vi "list_documents.vi"(0 "Device In":T1, 5 "error in":errorcluster) -> (14 "Device Out":T1, 15 "Comm":T2, 18 "Document list":string[][](array[string]), 19 "error out":errorcluster)   [LabVIEW 2019]
uses:
  <userlib>/IoT Devices/_subVIs/HTTPComm.ctl
  _SubVI/Cluster.ctl
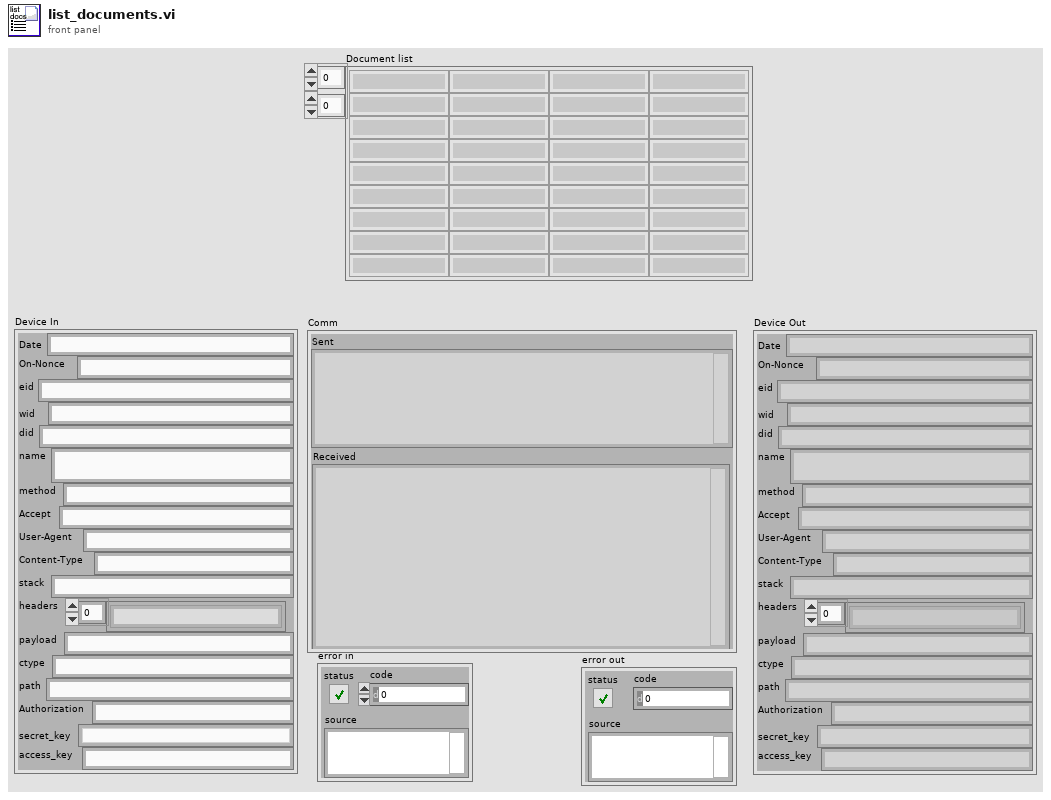
[diagram p1: front panel]
types:
  T1 = typedef "Cluster.ctl" = cluster{"Date":string, "On-Nonce":string, "eid":string, "wid":string, "did":string, "name":string, "method":string, "Accept":string, "User-Agent":string, "Content-Type":string, "stack":string, "headers":string[], "payload":string, "ctype":string, "path":string, "Authorization":string, "secret_key":string, "access_key":string}
  T2 = typedef "HTTPComm.ctl" = cluster{"url":string, "sent headers":string, "sent body":string, "headers":string, "body":string, "Sent":string, "Received":string}
  T3 = cluster{"items":cluster{"resourceType":string, "id":string, "name":string, "defaultWorkspace":cluster{"id":string}}[]}
  T4 = cluster{"resourceType":string, "id":string, "name":string, "defaultWorkspace":cluster{"id":string}}[]
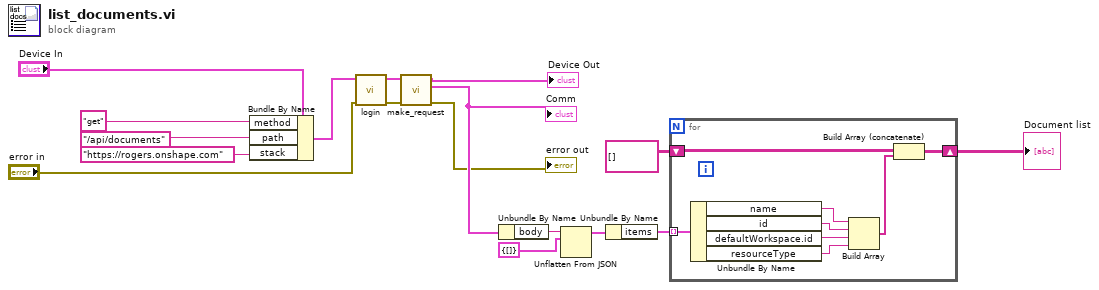
[diagram p0: block diagram]
diagram:
  n1 = Bundle By Name(cluster="Device In", "method"="get" ("Method"), "path"="/api/documents" ("payload"), "stack"="https://rogers.onshape.com" ("stacks")) -> (w5:T1)
  n2 = call "login.vi"("error in"="error in", "Device In"=w5) -> ("error out"=w6:errorcluster, "Device Out"=w4:T1)  [unwired: 8 in]
  n3 = call "make_request.vi"("Error in"=w6, "Device In"=w4) -> ("error out"=→"error out":errorcluster, "Comm"=w13:T2, "Device Out"=→"Device Out":T1)  [unwired: 7 in]
  "Comm" <- w13
  n4 = Unbundle By Name(w13) -> ("body"=w12:string)
  n5 = Unflatten From JSON(JSON string=w12, type and defaults=T3 {"items"=[]}) -> (value=w10:T3)  [unwired: 5 in, 1 out]
  n6 = Unbundle By Name(w10) -> ("items"=w9:T4)
  n7 = for {
    tunnel: w9 -> [w25] mode=indexing
    shift-right: [w23] -> w8
    shift-left: string[][] [] -> [w24]
    n8 = Unbundle By Name(w25) -> ("name"=w22:string, "id"=w21:string, "defaultWorkspace.id"=w20:string, "resourceType"=w18:string)
    n9 = Build Array(w22, w21, w20, w18) -> (w19:string[])
    n10 = Build Array (concatenate)(w24, w19) -> (w23:string[][])
  }
  "Document list" <- w8
